vi "Config Dev Point.vi"(8 "error in":errorcluster, 9 "Loss (0.0 jpF)":dbl min=-1900.0 max=19000.0 format="%#_10f", 10 "Capacitance (100.0 pF)":dbl=100.0 min=-165000.0 max=1650000.0 format="%#_10f", 11 "VISA resource name":refnum<visa-resource-name>) -> (0 "error out":errorcluster, 3 "VISA resource name out":refnum<visa-resource-name>)   [LabVIEW 2014, in "Andeen-Hagerling 2700.lvlib"]
doc: "This VI sets the capacitance and loss values for the Deviation Setpoint."
uses:
  Andeen-Hagerling 2700.lvlib
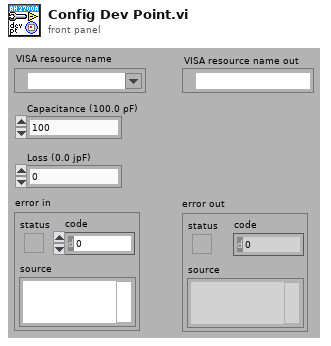
[diagram p1: front panel]
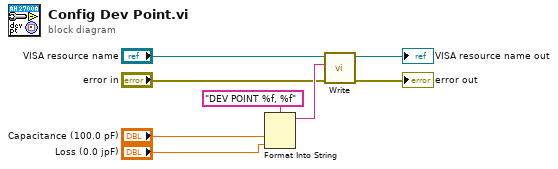
[diagram p0: block diagram]
diagram:
  n1 = Format Into String(format string="DEV POINT %f, %f", "Capacitance (100.0 pF)", "Loss (0.0 jpF)") -> (resulting string=w7:string)  [unwired: 2 in, 1 out]
  n2 = call "Write.vi"("error in"="error in", "command"=w7, "VISA resource name"="VISA resource name") -> ("error out"=→"error out":errorcluster, "VISA resource name out"=→"VISA resource name out":refnum<visa-resource-name>)  [unwired: 7 in]
